vi "Enable RT.vi"(7 "Virtual Memory Unit in":refnum<class "Virtual Memory Unit.lvclass">, 8 "error in (no error)":errorcluster, 11 "Remote Terminal in":refnum<class "Remote Terminal.lvclass">) -> (0 "error out":errorcluster, 3 "Remote Terminal out":refnum<class "Remote Terminal.lvclass">, 5 "Virtual Memory Unit out":refnum<class "Virtual Memory Unit.lvclass">)   [LabVIEW 2020, in "BCI-1553 API.lvlib" / "Remote Terminal.lvclass"]
doc: "Masks in the enable value for the Remote Terminal."
uses:
  Remote Terminal.lvclass
  Dependencies/Virtual Memory Unit/Virtual Memory Unit.lvclass
  Remote Terminal.lvclass/Remote Terminal.ctl
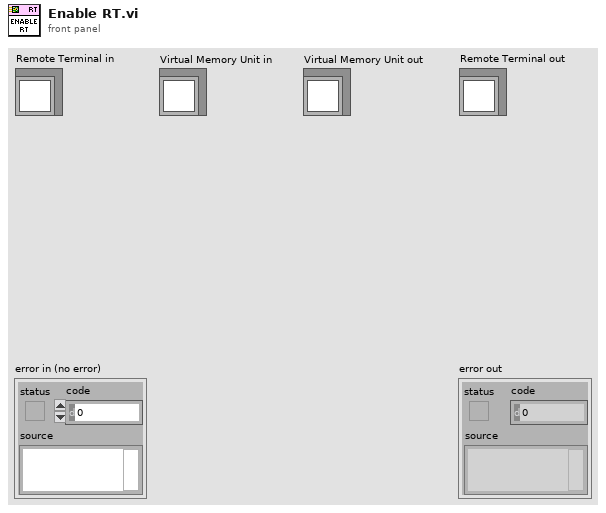
[diagram p1: front panel]
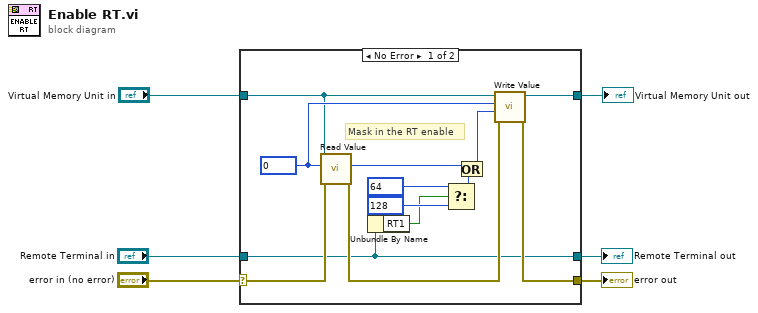
[diagram p0: block diagram]
diagram:
  n1 = case shown="No Error" "error in (no error)" {
    selector: "error in (no error)" -> [w12 w22]
    tunnel: [w10 w22] -> w5
    tunnel: [w9 w21] -> w3
    tunnel: "Remote Terminal in" -> [w9 w21]
    tunnel: "Virtual Memory Unit in" -> [w8 w20]
    tunnel: [w7 w20] -> w1
    frame No Error {
      w13 = 0 ("Address")
      # "Mask in the RT enable"
      n2 = call "Read Value.vi"("error in (no error)"=w12, "Index"=w13, "Virtual Memory Unit in"=w8) -> ("error out"=w11:errorcluster, "Value"=w19:u16)  [unwired: 7 in]
      n3 = Unbundle By Name(w9) -> ("RT1"=w16:bool)
      n4 = Select(t=u16 64 ("Address"), s=w16, f=u16 128 ("Address")) -> (s? t:f=w15:u16)
      n5 = Or(x=w19, y=w15) -> (x .or. y?=w14:u16)
      n6 = call "Write Value.vi"("error in (no error)"=w11, "Value"=w14, "Index"=w13, "Virtual Memory Unit in"=w8) -> ("error out"=w10:errorcluster, "Virtual Memory Unit out"=w7:refnum<class "Virtual Memory Unit.lvclass">)  [unwired: 6 in]
    }
    frame Error {
    }
  }
  "error out" <- w5
  "Remote Terminal out" <- w3
  "Virtual Memory Unit out" <- w1
